vi "HLine0003.vi"   [LabVIEW 2013]
uses:
  <vilib>/Heliosphere Research LLC/Advanced Plotting Toolkit/api_core/NewPlotType.ctl
  ModeType.ctl
  ErrorCodes.ctl
  <vilib>/Heliosphere Research LLC/Advanced Plotting Toolkit/Advanced Plotting Toolkit.lvlib
types:
  T1 = typedef "ErrorCodes.ctl" = u32
  T2 = typedef "ModeType.ctl" = enum16{"Normal", "Expected Failure", "Skipped", "Broken"}
  T3 = typedef "Advanced Plotting Toolkit.lvlib/NewPlotType.ctl" = enum16{"Rectangular Axes", "Polar Axes"}
  T4 = typedef "Advanced Plotting Toolkit.lvlib/PlotID.ctl" = i32
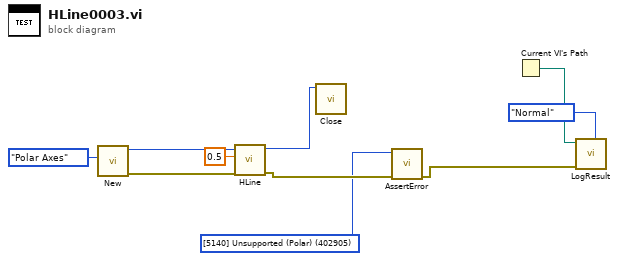
[diagram p0: block diagram]
diagram:
  w1 = T1 402905 items=["[5120] Invalid ID"=402902, "[5110] Failed to Init"=402900, "[5111] Unknown Error"=402901, "[5130] Save - Bad File Extension"=402403, "[5131] Save - General Error"=402904, "[5140] Unsupported (Polar)"=402905, "[5141] Unsupported (Logscale)"=402906, "[5142] Coordinates Not Regular"=402907] ("Expected Error")
  n1 = call <vilib>:"New.vi"("Plot Type"=NewPlotType."Polar Axes") -> ("error out"=w7:errorcluster, "Plot ID"=w8:T4)  [unwired: 9 in]
  n2 = call <vilib>:"HLine.vi"("error in (no error)"=w7, "Y (data coords)"=0.5, "Plot ID"=w8) -> ("error out"=w4:errorcluster, "Plot ID Out"=w2:T4)  [unwired: 7 in]
  n3 = call <vilib>:"Close.vi"("Plot ID"=w2) -> ()  [unwired: 10 in, 1 out]
  n4 = call "AssertError.vi"("error in (no error)"=w4, "Expected Error"=w1) -> ("error out"=w3:errorcluster)  [unwired: 9 in]
  n5 = Current VI's Path() -> (path=w10:path)
  n6 = call "LogResult.vi"("Mode"=ModeType."Normal", "Test Result"=w3, "VI Path"=w10) -> ()  [unwired: 9 in]
